vi "FM_Rx_Template.vi"() -> ()   [LabVIEW 2018]
uses:
  <vilib>/Analysis/3filter.llb/FIR Filter with I.C. (DBL).vi
  <instrlib>/niUSRP/niUSRP Fetch Rx Data (CDB WDT).vi
  <vilib>/Analysis/3filter.llb/Butterworth Filter (DBL).vi
  <vilib>/measure/maspectr.llb/FFT Power Spectrum and PSD for 1 Chan.vi
  <vilib>/Analysis/NI_AALPro.lvlib
  <vilib>/Analysis/NI_AALBase.lvlib
  <vilib>/measure/NI_MAPro.lvlib
panel:
  in  "Peak Deviation":i64=200000
  out "Demodulated Signal":waveform(dbl)(graph)
  out "Demodulated Signal Spectrum":cluster{"f0":dbl, "df":dbl, "magnitude":dbl[]}(graph)
  in  "stop":bool
  out "Error Out":errorcluster
  in  "Number of Samples":i64=200000
  in  "Active Antenna":string(combo)="RX2"
  out "Actual Gain (dB)":dbl format="%#_6f"
  in  "Gain (dB)":dbl format="%#_6f"
  out "Actual Frequency":dbl=100000.0 format="%#_6p"
  in  "Carrier Frequency":dbl=915000000.0 format="%#_6p"
  out "Actual IQ Rate":dbl=100000.0 format="%#_6p"
  in  "IQ Rate":dbl=1000000.0 format="%#_6p"
  in  "Device Names":refnum<k15>="192.168.10.2"
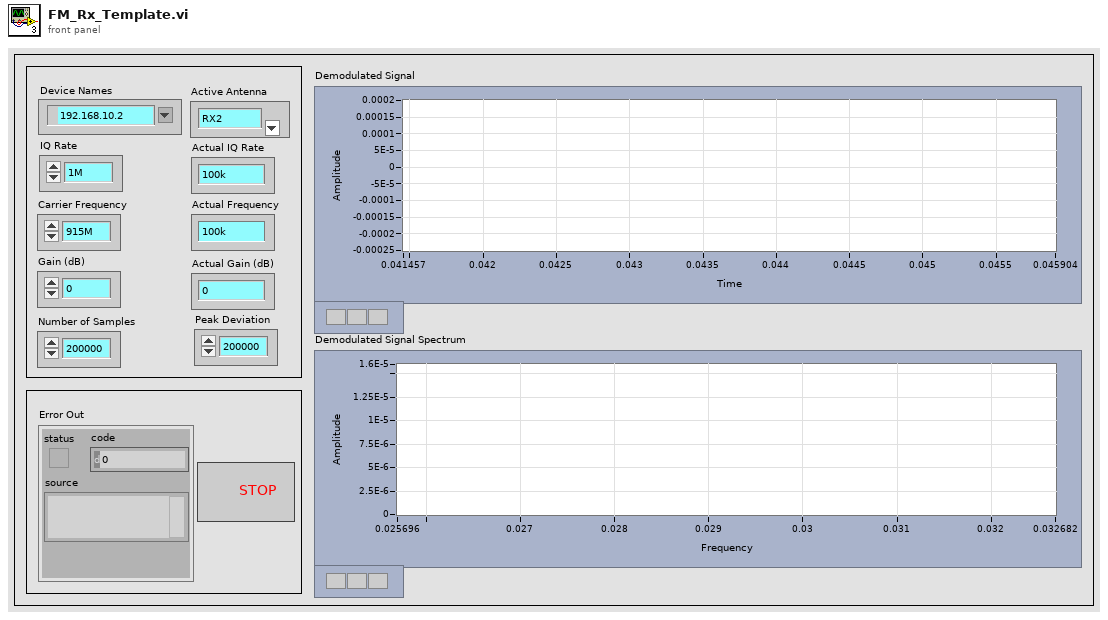
[diagram p1: front panel]
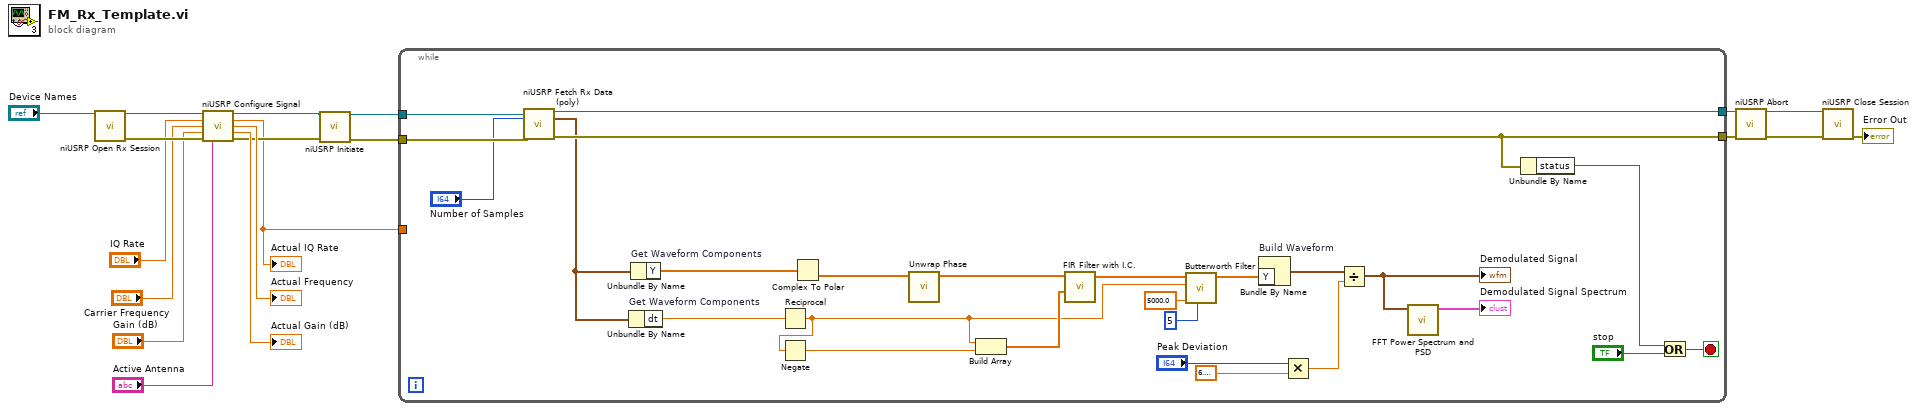
[diagram p0: block diagram]
diagram:
  n1 = call <instrlib>:"niUSRP Open Rx Session.vi"("device names"="Device Names") -> ("session handle out"=w18:refnum<k15>, "error out"=w17:errorcluster)  [unwired: 13 in]
  n2 = call <instrlib>:"niUSRP Configure Signal.vi"("session handle"=w18, "IQ rate"="IQ Rate", "carrier frequency"="Carrier Frequency", "gain"="Gain (dB)", "error in (no error)"=w17, "active antenna"="Active Antenna") -> ("session handle out"=w11:refnum<k15>, "coerced IQ rate"=w1:dbl, "coerced carrier frequency"=→"Actual Frequency":dbl, "coerced gain"=→"Actual Gain (dB)":dbl, "error out"=w10:errorcluster)  [unwired: 5 in]
  "Actual IQ Rate" <- w1
  n3 = call <instrlib>:"niUSRP Initiate.vi"("session handle"=w11, "error in (no error)"=w10) -> ("session handle out"=w8:refnum<k15>, "error out"=w7:errorcluster)  [unwired: 12 in]
  n4 = while {
    tunnel: w8 -> [w45]
    tunnel: w7 -> [w44]
    tunnel: [w43] -> w6
    tunnel: [w39] -> w5
    tunnel: w1 -> [_]
    stop <- w42 stop-if-true
    n5 = call-poly <instrlib>:"niUSRP Fetch Rx Data (poly).vi"("session handle"=w45, "number of samples"="Number of Samples", "error in (no error)"=w44) -> ("session handle out"=w43:refnum<k15>, "data"=w34:waveform(cdb), "error out"=w39:errorcluster)  [unwired: 9 in, 1 out]
    n6 = Unbundle By Name "Get Waveform Components"(w34) -> ("dt"=w33:dbl)
    n7 = Unbundle By Name "Get Waveform Components"(w34) -> ("Y"=w37:cdb[])
    n8 = Reciprocal(x=w33) -> (1/x=w29:dbl)
    n9 = Negate(x=w29) -> (-x=w32:dbl)
    n10 = Complex To Polar(r * e^(i*theta)=w37) -> (theta=w36:dbl[])  [unwired: 1 out]
    n11 = call <vilib>:"Unwrap Phase.vi"("Phase"=w36) -> ("Unwrapped Phase"=w35:dbl[])  [unwired: 9 in, 1 out]
    n12 = Build Array(w29, w32) -> (w31:dbl[])
    n13 = call-poly <vilib>:"FIR Filter with I.C..vi"("FIR Coefficients"=w31, "X"=w35) -> ("Filtered X"=w30:dbl[])  [unwired: 6 in, 2 out]
    n14 = call-poly <vilib>:"Butterworth Filter.vi"("order"=5, "low cutoff freq: fl"=5000.0, "sampling freq: fs"=w29, "X"=w30) -> ("Filtered X"=w26:dbl[])  [unwired: 4 in, 1 out]
    n15 = Bundle By Name "Build Waveform"("Y"=w26) -> (w25:waveform(dbl))  [unwired: 1 in]
    n16 = Multiply(x="Peak Deviation", y=6.283185307179586) -> (x*y=w22:dbl)
    n17 = Divide(x=w25, y=w22) -> (x/y=w21:waveform(dbl))
    "Demodulated Signal" <- w21
    n18 = call-poly <vilib>:"FFT Power Spectrum and PSD.vi"("time signal"=w21) -> ("Power Spectrum / PSD"=→"Demodulated Signal Spectrum":cluster{"f0":dbl, "df":dbl, "magnitude":dbl[]})  [unwired: 7 in, 3 out]
    n19 = Unbundle By Name(w39) -> ("status"=w41:bool)
    n20 = Or(x=w41, y="stop") -> (x .or. y?=w42:bool)
  }
  n21 = call <instrlib>:"niUSRP Abort.vi"("session handle"=w6, "error in (no error)"=w5) -> ("session handle out"=w4:refnum<k15>, "error out"=w3:errorcluster)  [unwired: 12 in]
  n22 = call <instrlib>:"niUSRP Close Session.vi"("session handle"=w4, "error in (no error)"=w3) -> ("error out"=→"Error Out":errorcluster)  [unwired: 13 in]
